vi "Get State.vi"(8 "error in (no error)":errorcluster, 11 "Command in":refnum<class "Drive by Power.lvclass">) -> (0 "error out":errorcluster, 1 "Command State String":string, 3 "Command out":refnum<class "Drive by Power.lvclass">)   [LabVIEW 2014, in "Forward Drive.lvlib" / "Drive by Power.lvclass"]
uses:
  Drive by Power.lvclass
  Forward Drive Cmd.lvclass
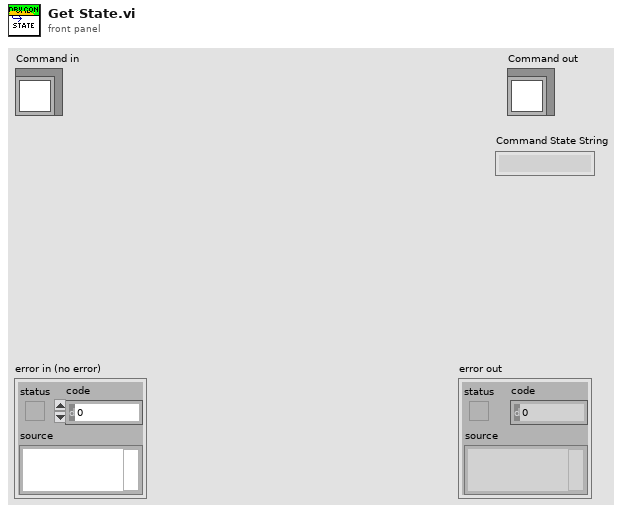
[diagram p1: front panel]
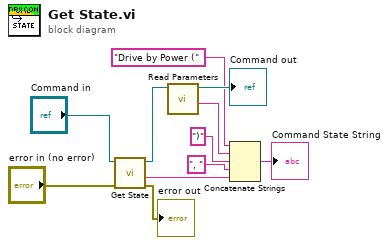
[diagram p0: block diagram]
diagram:
  n1 = call-parent "Get State.vi"("error in (no error)"="error in (no error)", "Command in"="Command in") -> ("error out"=→"error out":errorcluster, "Command State String"=w4:string, "Command out"=w8:refnum<class "Drive by Power.lvclass">)  [unwired: 7 in]
  n2 = call-dynamic "Read Parameters.vi"("Drive by Power in"=w8) -> ("Parameters String"=w5:string, "Drive by Power out"=→"Command out":refnum<class "Drive by Power.lvclass">)  [unwired: 7 in, 2 out]
  n3 = Concatenate Strings("Drive by Power (" ("string"), w5, ")" ("string"), ", " ("string"), w4) -> (→"Command State String":string)
